vi "Populate Font ComboBox.vi"(8 "error in":errorcluster, 9 "Font in":string, 11 "CmbBox Refnum":refnum<vi>) -> (0 "error out":errorcluster, 1 "Font out":string)   [LabVIEW 2012]
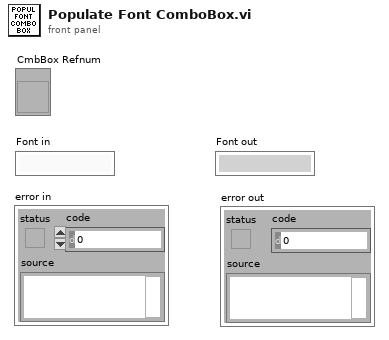
[diagram p1: front panel]
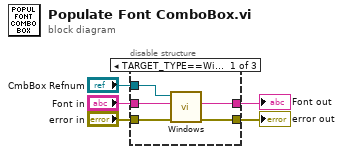
[diagram p0: block diagram]
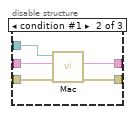
[diagram p2: hidden frame]
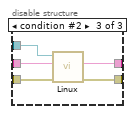
[diagram p3: hidden frame]
diagram:
  n1 = disable-structure shown="TARGET_TYPE==Windows, default" {
    disable-tunnel: "CmbBox Refnum" -> [w10 w15 w18]
    disable-tunnel: "error in" -> [w9 w14 w20]
    disable-tunnel: [w8 w13 w19] -> w5
    disable-tunnel: "Font in" -> [w7 w12 w17]
    disable-tunnel: [w6 w11 w16] -> w1
    frame condition #0 (active) {
      n2 = call <resource>:"Windows.vi"("error in (no error)"=w9, "Font in"=w7, "Font"=w10) -> ("error out"=w8:errorcluster, "Font out"=w6:string)  [unwired: 7 out]
    }
    frame condition #1 {
      n3 = call <resource>:"Mac.vi"("error in (no error)"=w14, "Font in"=w12, "Font"=w15) -> ("error out"=w13:errorcluster, "Font out"=w11:string)  [unwired: 7 in]
    }
    frame condition #2 {
      n4 = call <resource>:"Linux.vi"("error in (no error)"=w20, "Font in"=w17, "Font"=w18) -> ("error out"=w19:errorcluster, "Font out"=w16:string)  [unwired: 7 in]
    }
  }
  "error out" <- w5
  "Font out" <- w1
